vi "Tell Child Init.vi"(6 "Alias":string, 7 "Actor in":refnum<class "Actor.lvclass">, 8 "Error in":errorcluster, 10 "Input":T1) -> (0 "Error out":errorcluster, 5 "Actor out":refnum<class "Actor.lvclass">)   [LabVIEW 2020, in "_Template.lvlib" / "Templates.lvlib" / "TEMPLATE jettl Msg.lvlib" / "TEMPLATE.lvlib"]
uses:
  TEMPLATE.lvlib
  jettl/jettl/jettl.lvlib
  TEMPLATE jettl Msg.lvlib
  jettl/jettl/Actor/Actor.lvclass
  Input.ctl
panel:
  # "This front panel should not be manipulated."
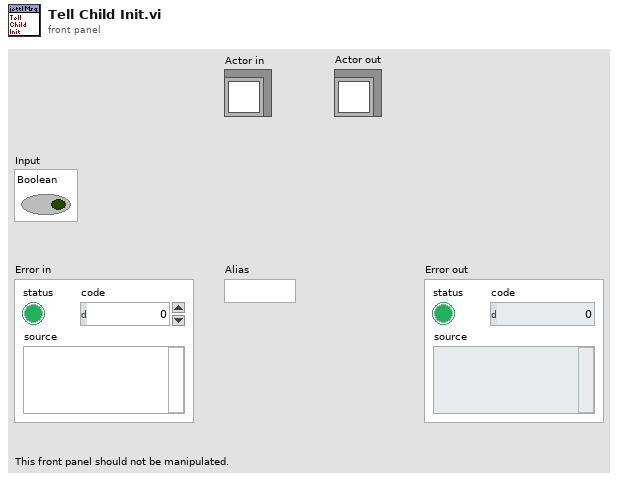
[diagram p1: front panel]
types:
  T1 = typedef "_Template.lvlib/Templates.lvlib/TEMPLATE jettl Msg.lvlib/Input.ctl" = cluster{"Boolean":bool}
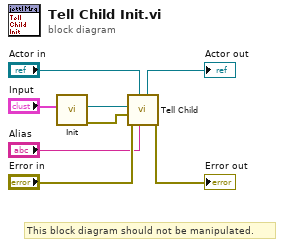
[diagram p0: block diagram]
diagram:
  # "This block diagram should not be manipulated."
  n1 = call "Init.vi"("Input"="Input") -> ("Error out"=w2:errorcluster, "Msg Attributes"=w4:refnum<data-value>)  [unwired: 9 in]
  n2 = call "Tell Child.vi"("Alias"="Alias", "Actor in"="Actor in", "Error in"="Error in", "Error"=w2, "Msg Attributes"=w4) -> ("Error out"=→"Error out":errorcluster, "Actor out"=→"Actor out":refnum<class "Actor.lvclass">)  [unwired: 5 in]
